vi "SWITCH Configure Filter.vi"(8 "error in (no error)":errorcluster, 10 "Message Data":variant, 11 "Data Cluster in":T1={"Tango HW"={"VISA resource"="101:110", "Baud Rate (115200)"=0, "lAnInterfaceType"=0, "bAShowProt"=0}, "Writer Queue"=refnum, "Status"=FALSE, "Abs Position"=[], "Axis Velocity"={"dX"=0.0, "dY"=0.0, "dZ"=0.0, "dA"=0.0}, "acceleration "=0.0, "Z direction"=enum."Up", "Position Mode"="", "plLSID"=0}) -> (0 "error out":errorcluster, 3 "Data Cluster out":T1={"Tango HW"={"VISA resource"="101:110", "Baud Rate (115200)"=0, "lAnInterfaceType"=0, "bAShowProt"=0}, "Writer Queue"=refnum, "Status"=FALSE, "Abs Position"=[], "Axis Velocity"={"dX"=0.0, "dY"=0.0, "dZ"=0.0, "dA"=0.0}, "acceleration "=0.0, "Z direction"=enum."Up", "Position Mode"="", "plLSID"=0})   [LabVIEW 2020, in "MOTOR.lvlib"]
uses:
  MOTOR.lvlib
  support/Message Queue/Message Cluster.ctl
  support/Message Queue/Message Queue.lvlib
  support/HW Message Cluster.ctl
  PS Hardware Configuration.ctl
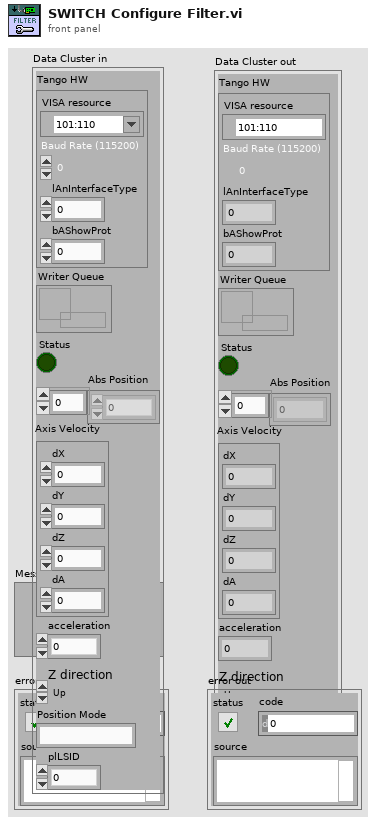
[diagram p1: front panel]
types:
  T1 = typedef "MOTOR.lvlib/PS Hardware Configuration.ctl" = cluster{"Tango HW":cluster{"VISA resource":refnum<visa-resource-name>, "Baud Rate (115200)":i32, "lAnInterfaceType":i32, "bAShowProt":i32}, "Writer Queue":refnum<queue>, "Status":bool, "Abs Position":i32[], "Axis Velocity":cluster{"dX":dbl, "dY":dbl, "dZ":dbl, "dA":dbl}, "acceleration ":dbl, "Z direction":enum16{"Up", "Down"}, "Position Mode":string, "plLSID":i32}
  T2 = cluster{"Scan List":string, "Filter Window (%) (0.1)":dbl, "Filter Count (10)":i32, "Filter Type (0:Off)":u16}
  T3 = typedef "Message Queue.lvlib/HW Message Cluster.ctl" = cluster{"Writer Queue":refnum<queue>, "Writer Data":T4}
  T4 = typedef "Message Queue.lvlib/Message Cluster.ctl" = cluster{"Message":string, "Message Data":variant}
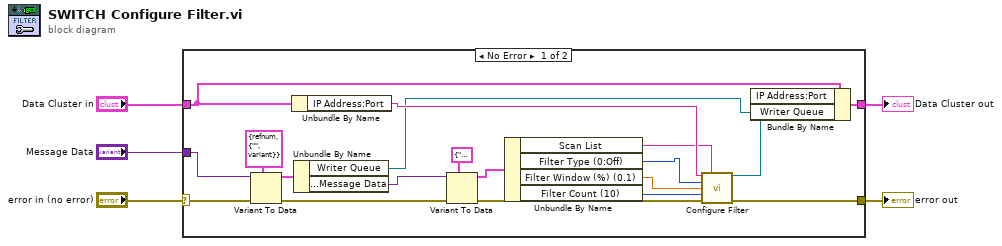
[diagram p0: block diagram]
diagram:
  n1 = case shown="No Error" "error in (no error)" {
    selector: "error in (no error)" -> [w16 w25]
    tunnel: "Message Data" -> [w14 _]
    tunnel: [w24 w26] -> w4
    tunnel: "Data Cluster in" -> [w23 w26]
    tunnel: [w19 w25] -> w2
    frame No Error {
      n2 = Variant To Data(error in=w16, type=T3 {"Writer Queue"=refnum, "Writer Data"={"Message"="", "Message Data"=variant}}, Variant=w14) -> (data=w17:T3, error out=w15:errorcluster)
      n3 = Unbundle By Name(w23) -> ("IP Address:Port"=w21:string)
      n4 = Unbundle By Name(w17) -> ("Writer Queue"=w12:refnum<queue>, "Writer Data.Message Data"=w13:variant)
      n5 = Variant To Data(error in=w15, type=T2 {"Scan List"="1", "Filter Window (%) (0.1)"=0.1, "Filter Count (10)"=10, "Filter Type (0:Off)"=0}, Variant=w13) -> (data=w22:T2, error out=w18:errorcluster)
      n6 = Unbundle By Name(w22) -> ("Scan List"=w11:string, "Filter Type (0:Off)"=w8:u16, "Filter Window (%) (0.1)"=w7:dbl, "Filter Count (10)"=w6:i32)
      n7 = call <vilib>:"Configure Filter.vi"("VISA resource name"=w21, "Scan List (Empty)"=w11, "Filter Type (0:Off)"=w8, "Filter Window (%) (0.1)"=w7, "Filter Count (10)"=w6, "error in (no error)"=w18) -> ("VISA resource name out"=w20:refnum<visa-resource-name>, "error out"=w19:errorcluster)  [unwired: 8 in]
      n8 = Bundle By Name(cluster=w23, "IP Address:Port"=w20, "Writer Queue"=w12) -> (w24:T1)
    }
    frame Error {
    }
  }
  "Data Cluster out" <- w4
  "error out" <- w2
